vi "override timing.vi"(6 "Priority":u64, 8 "error in (no error)":errorcluster, 9 "Offset":u64, 10 "Decimation":u64=1, 11 "Mock Transfer Group in":refnum<class "Mock Transfer Group.lvclass">) -> (0 "error out":errorcluster, 3 "Mock Transfer Group out":refnum<class "Mock Transfer Group.lvclass">)   [LabVIEW 2017, in "Mock Transfer Group.lvclass"]
uses:
  Mock Transfer Group.lvclass
  C:/github/data-sharing-framework/Data Sharing Framework Core/Engine/Classes/Transfer Group/Transfer Group.lvclass
  Engine/Classes/Transfer Group/Transfer Group.lvclass/Transfer Group.ctl
  Engine/Classes/Transfer Group/Transfer Group.lvclass
  Engine/Classes/Timing/Timing.lvclass
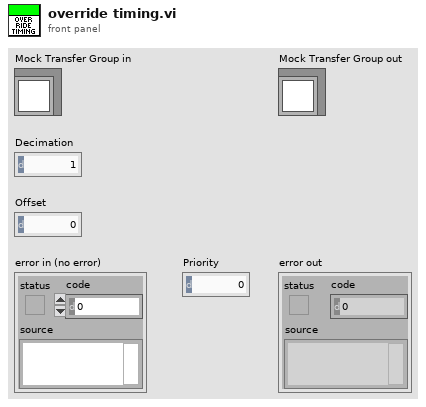
[diagram p1: front panel]
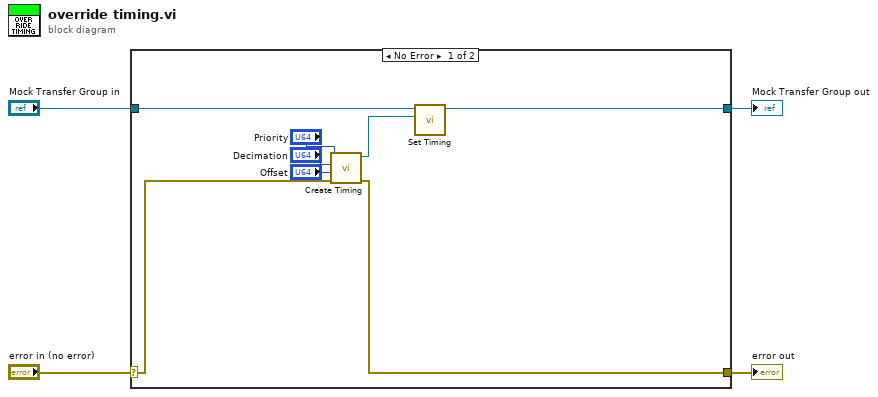
[diagram p0: block diagram]
diagram:
  n1 = case shown="No Error" "error in (no error)" {
    selector: "error in (no error)" -> [w9 w14]
    tunnel: [w8 w14] -> w3
    tunnel: [w11 w13] -> w1
    tunnel: "Mock Transfer Group in" -> [w12 w13]
    frame No Error {
      n2 = call "Create Timing.vi"("error in (no error)"=w9, "Offset"="Offset", "Decimation"="Decimation", "Priority"="Priority") -> ("error out"=w8:errorcluster, "Timing"=w10:refnum<class "Timing.lvclass">)  [unwired: 6 in]
      n3 = call "Set Timing.vi"("Timing"=w10, "Transfer Group in"=w12) -> ("Transfer Group out"=w11:refnum<class "Mock Transfer Group.lvclass">)  [unwired: 9 in]
    }
    frame Error {
    }
  }
  "error out" <- w3
  "Mock Transfer Group out" <- w1
